vi "Update Value.vi"(6 "Time":dbl, 8 "error in (no error)":errorcluster, 11 "BluelinesRedlines in":refnum<class "BluelinesRedlines.lvclass">) -> (0 "error out":errorcluster, 1 "Update":bool, 2 "Value":variant, 3 "BluelinesRedlines out":refnum<class "BluelinesRedlines.lvclass">)   [LabVIEW 2020, in "VolatusGUIElements.lvlib" / "BluelinesRedlines.lvclass"]
uses:
  BluelinesRedlines.lvclass
  BluelinesRedlines.lvclass/BluelinesRedlines.ctl
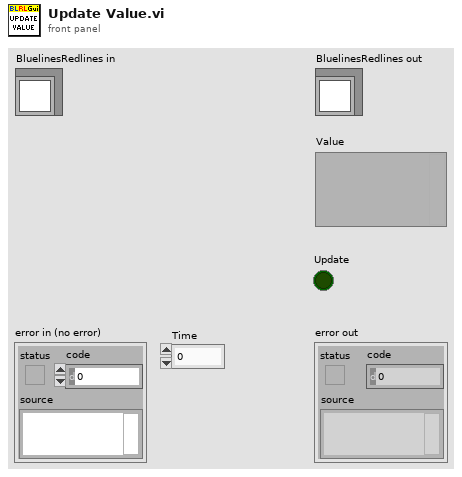
[diagram p1: front panel]
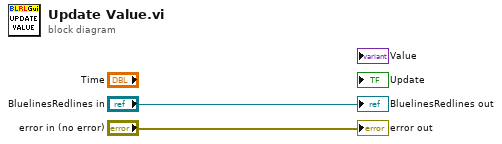
[diagram p0: block diagram]
diagram:
  "error out" <- "error in (no error)"
  "BluelinesRedlines out" <- "BluelinesRedlines in"
